vi "PopulateExposureTime.vi"(10 "Exposure Time":refnum<vi>, 11 ".NET Refnum in":refnum<k24>) -> ()   [LabVIEW 2019]
uses:
  Dependencies/PVCamNET.dll
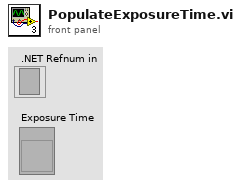
[diagram p1: front panel]
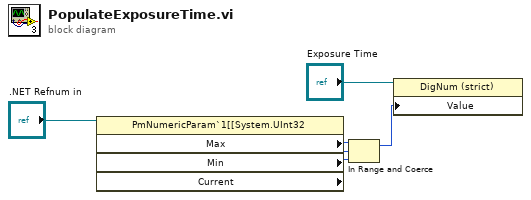
[diagram p0: block diagram]
diagram:
  n1 = property class="PmNumericParam`1[[System.UInt32"(reference=".NET Refnum in") -> ("Max"=w2:u32, "Min"=w3:u32, "Current"=w4:u32)  [unwired: 1 in, 2 out]
  n2 = In Range and Coerce(upper limit=w2, x=w4, lower limit=w3) -> (coerced(x)=w6:u32)  [unwired: 1 out]
  n3 = property class="DigNum (strict)"(reference="Exposure Time", "Value"=w6) -> ()  [unwired: 1 in, 2 out]
